vi "Is Cooler On.vi"(8 "error in (no error)":errorcluster, 11 "iCoolerStatus":i32) -> (0 "error out":errorcluster, 2 "function return":u32, 3 "iCoolerStatus out":i32)   [LabVIEW 2018, in "AndorSDK.lvlib"]
doc: "EXPNETTYPE unsigned int WINAPI IsCoolerOn(int * iCoolerStatus);"
uses:
  AndorSDK.lvlib
  ATMCD32D.dll
  OwnVIs/AndorOWN.lvlib
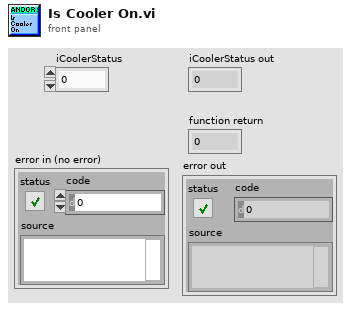
[diagram p1: front panel]
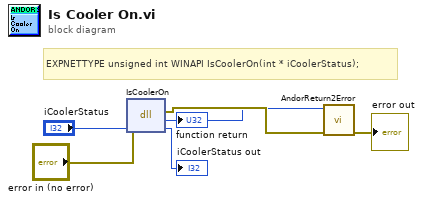
[diagram p0: block diagram]
diagram:
  # "EXPNETTYPE unsigned int WINAPI IsCoolerOn(int * iCoolerStatus);"
  n1 = dll-call lib="C:/Users/e14user/Documents/LabVIEW software/GitRepo/lib/ANDOR/Andor SDK/ATMCD32D.*" fn="IsCoolerOn"(error in="error in (no error)", "iCoolerStatus"="iCoolerStatus") -> (error out=w3:errorcluster, w2:u32, "iCoolerStatus"=→"iCoolerStatus out":i32)  [unwired: 2 in, 1 out]
  "function return" <- w2
  n2 = call "AndorReturn2Error.vi"("error in (no error)"=w3, "Camera return"=w2) -> ("error out"=→"error out":errorcluster)  [unwired: 9 in]
